vi "Forcade_ZoomPictureSize.vi"(8 "error in (no error)":errorcluster caption="错误输入（无错误）", 9 "Origin":T1, 10 "Bounds":T3, 11 "Picture_Class 输入":refnum<class "Picture_Class.lvclass"> caption="DNL_LabVIEW Object in") -> (0 "error out":errorcluster caption="错误输出", 1 "2D Picture Out":picture, 2 "Image Data":T2, 3 "Picture_Class 输出":refnum<class "Picture_Class.lvclass"> caption="DNL_LabVIEW Object out")   [LabVIEW 2013, in "Picture_Class.lvclass"]
uses:
  Picture_Class.lvclass
  <vilib>/Utility/miscctls.llb/LVBoundsTypeDef.ctl
  <vilib>/picture/picture.llb/imagedata.ctl
  <vilib>/Utility/miscctls.llb/LVPoint32TypeDef.ctl
  Picture_Class.lvclass/Picture_Class.ctl
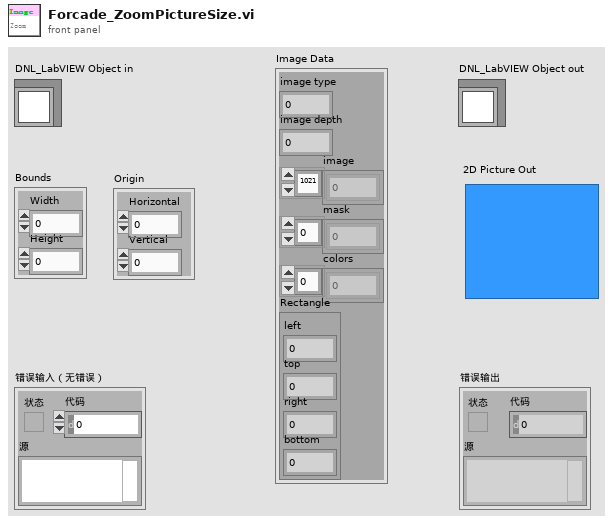
[diagram p1: front panel]
types:
  T1 = typedef "LVPoint32TypeDef.ctl" = cluster{"Horizontal":i32, "Vertical":i32}
  T2 = typedef "imagedata.ctl" = cluster{"image type":i32, "image depth":i32, "image":u8[], "mask":u8[], "colors":u32[], "Rectangle":cluster{"left":i16, "top":i16, "right":i16, "bottom":i16}}
  T3 = typedef "LVBoundsTypeDef.ctl" = cluster{"Width":u32, "Height":u32}
  T4 = cluster{"left":i16, "top":i16, "right":i16, "bottom":i16}
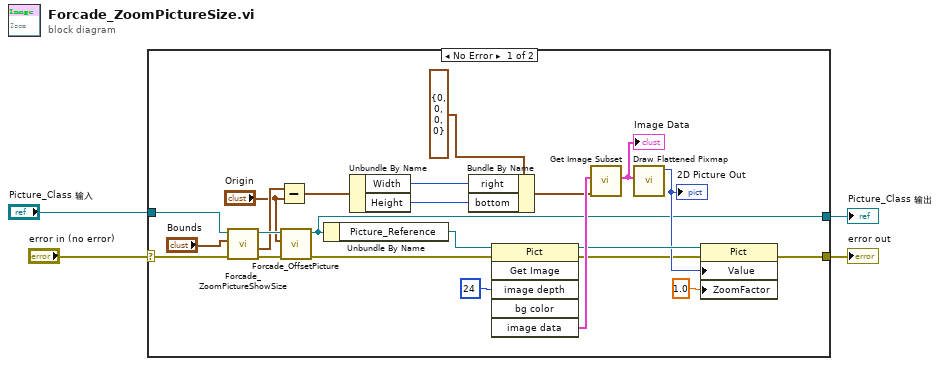
[diagram p0: block diagram]
diagram:
  n1 = case shown="No Error" "error in (no error)" {
    selector: "error in (no error)" -> [w22 w29]
    tunnel: [w11 w29] -> w3
    tunnel: [w9 w28] -> w1
    tunnel: "Picture_Class 输入" -> [w27 w28]
    frame No Error {
      n2 = call "Forcade_ZoomPictureShowSize.vi"("error in (no error)"=w22, "Bounds"="Bounds", "Picture_Class 输入"=w27) -> ("error out"=w8:errorcluster, "RealSize"=w16:T3, "Picture_Class 输出"=w23:refnum<class "Picture_Class.lvclass">)  [unwired: 5 in, 1 out]
      n3 = Subtract(x=w16, y="Origin") -> (x-y=w6:T3)
      n4 = call "Forcade_OffsetPicture.vi"("error in (no error)"=w8, "Origin"="Origin", "Picture_Class 输入"=w23) -> ("error out"=w7:errorcluster, "Picture_Class 输出"=w9:refnum<class "Picture_Class.lvclass">)  [unwired: 7 in]
      n5 = Unbundle By Name(w9) -> ("Picture_Reference"=w24:refnum<vi>)
      n6 = Unbundle By Name(w6) -> ("Width"=w18:u32, "Height"=w17:u32)
      n7 = Bundle By Name(cluster=T4 {"left"=0, "top"=0, "right"=0, "bottom"=0} ("subset rect"), "right"=w18, "bottom"=w17) -> (w15:T4)
      n8 = invoke on="Invoke Node" class="Pict" method="Get Image"(reference=w24, error in=w7, "image depth"=24 ("Image Depth")) -> (reference out=w14:refnum<vi>, error out=w12:errorcluster, "image data"=w21:T2)  [unwired: 3 in, 3 out]
      n9 = call <vilib>:"Get Image Subset.vi"("subset rect"=w15, "image data"=w21) -> ("image subset"=w20:T2)  [unwired: 4 in, 1 out]
      "Image Data" <- w20
      n10 = call <vilib>:"Draw Flattened Pixmap.vi"("image data"=w20) -> ("new picture"=w13:picture)  [unwired: 8 in]
      "2D Picture Out" <- w13
      n11 = property class="Pict"(reference=w14, error in=w12, "Value"=w13, "ZoomFactor"=sgl 1.0 ("Zoom Factor")) -> (error out=w11:errorcluster)  [unwired: 1 out]
    }
    frame Error {
    }
  }
  "error out" <- w3
  "Picture_Class 输出" <- w1
